vi "Invert bit stream.vi"(11 "normal":u8[](array[numeric])) -> (3 "inverted":u8[](array[numeric]))   [LabVIEW 2019]
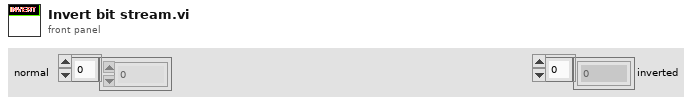
[diagram p1: front panel]
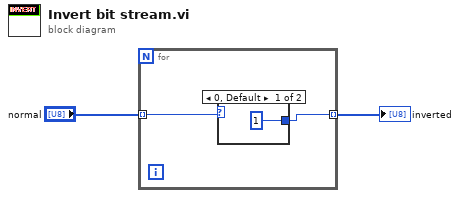
[diagram p0: block diagram]
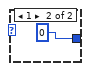
[diagram p2: hidden frame]
diagram:
  n1 = for {
    tunnel: "normal" -> [w4] mode=indexing
    tunnel: [w3] -> w1 mode=indexing
    n2 = case shown="0, Default" w4 {
      tunnel: [u8 1 ("Numeric") u8 0 ("Numeric")] -> w3
      frame 0, Default {
      }
      frame 1 {
      }
    }
  }
  "inverted" <- w1
